vi "transfer function.vi"() -> ()   [LabVIEW 2016]
uses:
  <vilib>/DAQmx/write.llb/DAQmx Write (Analog Wfm 1Chan NSamp).vi
  <vilib>/DAQmx/read.llb/DAQmx Read (Analog Wfm 1Chan NSamp).vi
  <vilib>/DAQmx/create/channels.llb/DAQmx Create Channel (AO-Voltage-Basic).vi
  <vilib>/DAQmx/create/channels.llb/DAQmx Create Channel (AI-Voltage-Basic).vi
  <vilib>/DAQmx/configure/timing.llb/DAQmx Timing (Sample Clock).vi
  <vilib>/DAQmx/miscellaneous.llb/DAQmx Fill In Error Info.vi
  <vilib>/DAQmx/configure/trigger.llb/DAQmx Start Trigger (Digital Edge).vi
  <vilib>/Waveform/WDTFileIO.llb/Export Waveforms To Spreadsheet File (1D).vi
  <vilib>/measure/NI_MABase.lvlib
  <resource>/objmgr/daqmx.rc
panel:
  in  "File Name":string
  in  "Number of steps":i32
  in  "frequency stop":dbl=10.0 format="%0.2p"
  in  "file path (dialog if empty)":path
  out "Waveform Graph 2":waveform(dbl)(graph)
  in  "number of periods":dbl
  in  "amplitude":dbl=1.0 format="%0.2p"
  in  "frequency start":dbl=10.0 format="%0.2p"
  out "Waveform Graph":waveform(dbl)[](graph)
  out "number of samples written per channel":u32
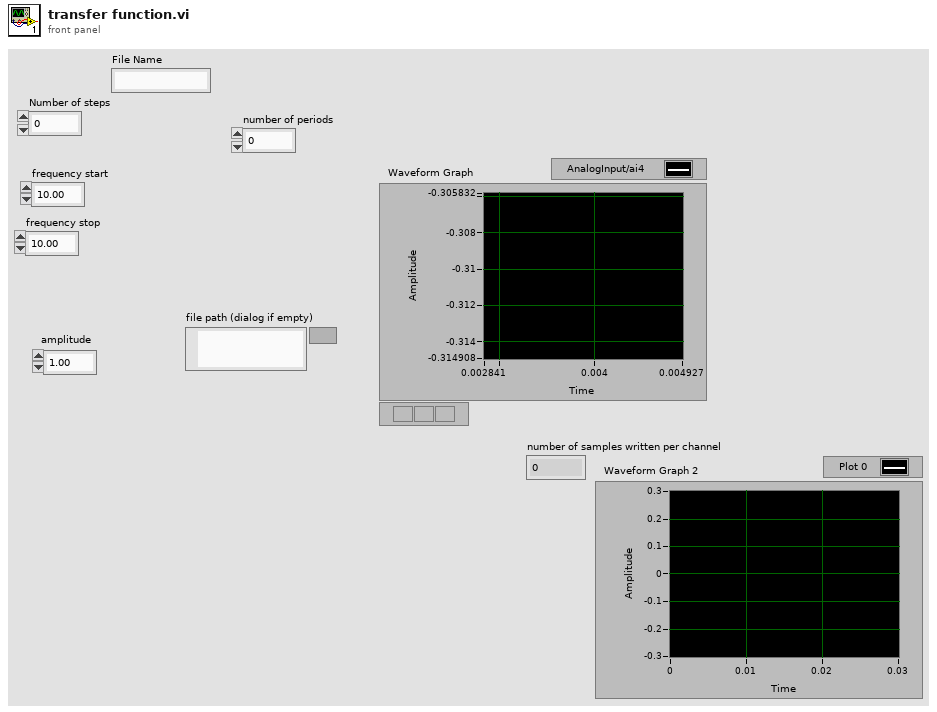
[diagram p1: front panel]
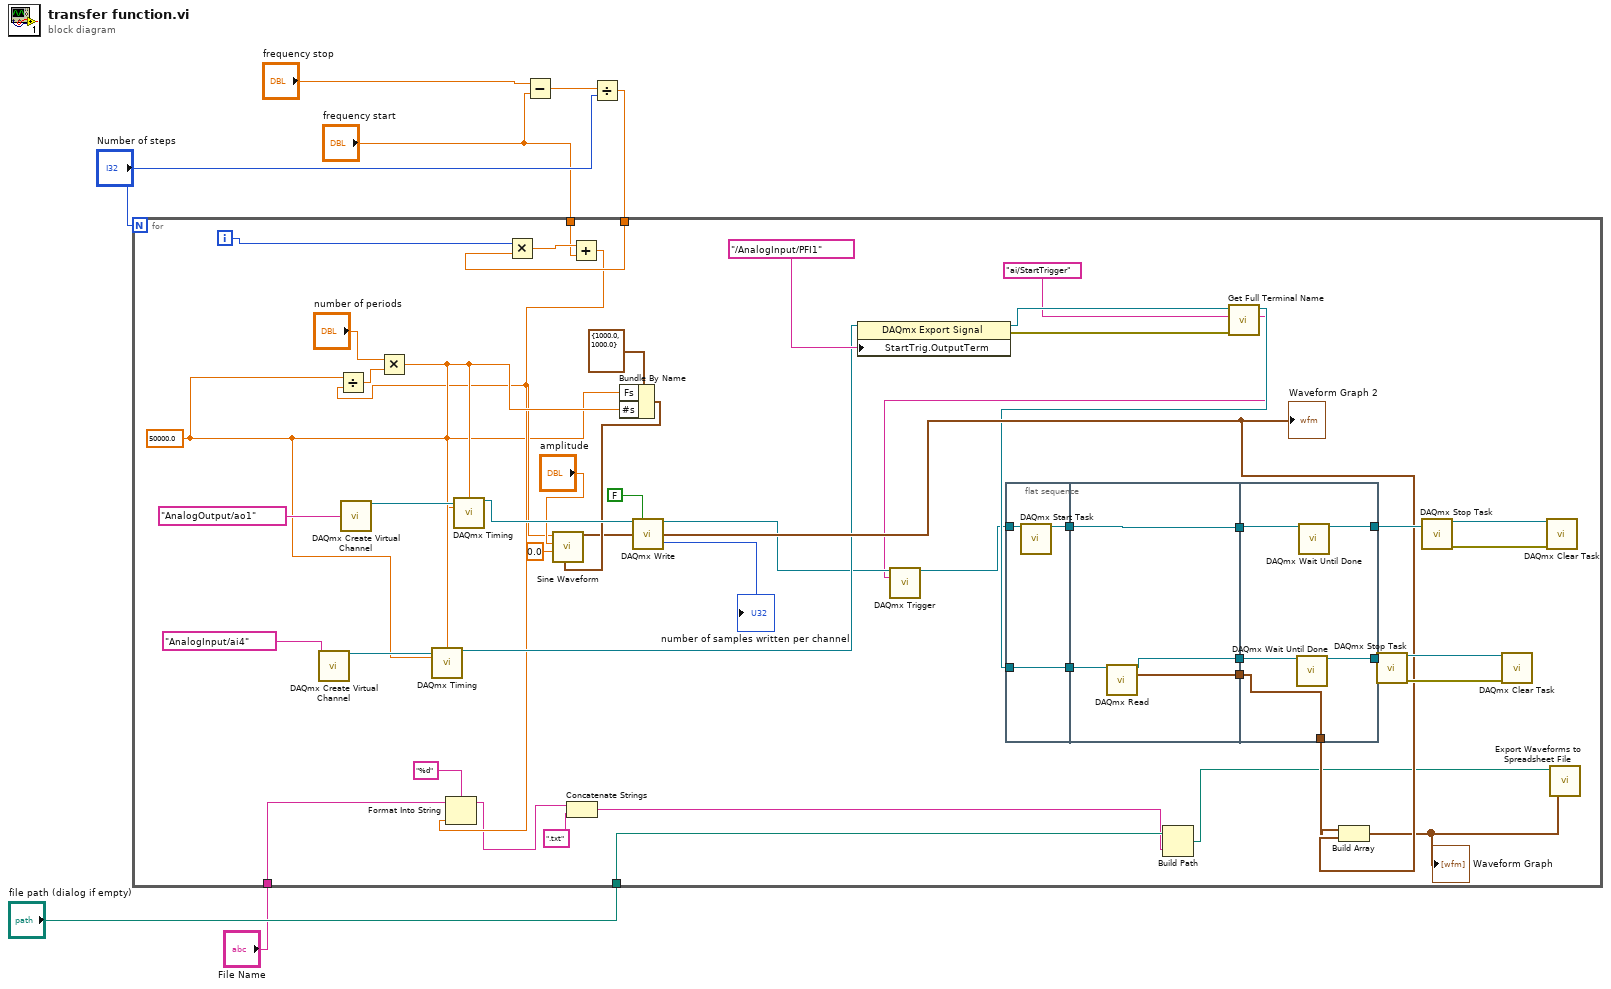
[diagram p0: block diagram]
diagram:
  n1 = Subtract(x="frequency stop", y="frequency start") -> (x-y=w7:dbl)
  n2 = Divide(x=w7, y="Number of steps") -> (x/y=w5:dbl)
  n3 = for {
    N: "Number of steps" -> [_]
    tunnel: w5 -> [w19]
    tunnel: "frequency start" -> [w17]
    tunnel: "file path (dialog if empty)" -> [w16]
    tunnel: "File Name" -> [w15]
    i -> [w20]
    w8 = 50000.0 ("rate")
    n4 = call-poly <vilib>:"DAQmx Create Virtual Channel.vi"("physical channels"=tag "AnalogInput/ai4") -> ("task out"=w45:refnum<k21>)  [unwired: 13 in, 1 out]
    n5 = call-poly <vilib>:"DAQmx Create Virtual Channel.vi"("physical channels"=tag "AnalogOutput/ao1") -> ("task out"=w50:refnum<k21>)  [unwired: 13 in, 1 out]
    n6 = Multiply(x=w20, y=w19) -> (x*y=w18:dbl)
    n7 = Add(x=w18, y=w17) -> (x+y=w14:dbl)
    n8 = Divide(x=w8, y=w14) -> (x/y=w37:dbl)
    n9 = Multiply(x="number of periods", y=w37) -> (x*y=w34:dbl)
    n10 = call-poly <vilib>:"DAQmx Timing.vi"("task/channels in"=w45, "samples per channel"=w34, "rate"=w8) -> ("task out"=w27:refnum<k21>)  [unwired: 11 in, 1 out]
    n11 = Format Into String(format string="%d", initial string=w15, w14) -> (resulting string=w11:string)  [unwired: 1 in, 1 out]
    n12 = call-poly <vilib>:"DAQmx Timing.vi"("task/channels in"=w50, "samples per channel"=w34, "rate"=w8) -> ("task out"=w49:refnum<k21>)  [unwired: 11 in, 1 out]
    n13 = Concatenate Strings(w11, ".txt" ("string")) -> (w10:string)
    n14 = Bundle By Name(cluster=cluster{"Fs":dbl, "#s":dbl} {"Fs"=1000.0, "#s"=1000.0} ("sampling info"), "Fs"=w8, "#s"=w34) -> (w35:cluster{"Fs":dbl, "#s":dbl})
    n15 = call <vilib>:"Sine Waveform.vi"("sampling info"=w35, "phase"=0.0, "amplitude"="amplitude", "frequency"=w14) -> ("signal out"=w32:waveform(dbl))  [unwired: 6 in, 1 out]
    "Waveform Graph 2" <- w32
    n16 = call-poly <vilib>:"DAQmx Write.vi"("task/channels in"=w49, "auto start"=FALSE, "data"=w32) -> ("task out"=w25:refnum<k21>, "number of samples written per channel"=→"number of samples written per channel":u32)  [unwired: 10 in, 1 out]
    n17 = property class="DAQmx Export Signal"(reference=w27, "StartTrig.OutputTerm"=tag "/AnalogInput/PFI1") -> (reference out=w29:refnum<k21>, error out=w30:errorcluster)  [unwired: 1 in]
    n18 = flat-sequence {
      tunnel: w24 -> [w60]
      tunnel: [w59] -> w57
      tunnel: w26 -> [w58]
      tunnel: [w58] -> w56
      tunnel: w57 -> [w64]
      tunnel: w56 -> [w63]
      tunnel: [w64] -> w55
      tunnel: [w62] -> w54
      tunnel: [w61] -> w53
      tunnel: w55 -> [w69]
      tunnel: [w68] -> w43
      tunnel: [w67] -> w40
      tunnel: w54 -> [w66]
      tunnel: [w65] -> w33
      tunnel: w53 -> [w65]
      frame #0 {
        n19 = call <vilib>:"DAQmx Start Task.vi"("task/channels in"=w60) -> ("task out"=w59:refnum<k21>)  [unwired: 13 in, 1 out]
      }
      frame #1 {
        n20 = call-poly <vilib>:"DAQmx Read.vi"("task/channels in"=w63) -> ("task out"=w62:refnum<k21>, "data"=w61:waveform(dbl))  [unwired: 12 in, 1 out]
      }
      frame #2 {
        n21 = call <vilib>:"DAQmx Wait Until Done.vi"("task/channels in"=w66) -> ("task out"=w67:refnum<k21>)  [unwired: 13 in, 1 out]
        n22 = call <vilib>:"DAQmx Wait Until Done.vi"("task/channels in"=w69) -> ("task out"=w68:refnum<k21>)  [unwired: 13 in, 1 out]
      }
    }
    n23 = Build Path(base path=w16, name or relative path=w10) -> (appended path=w13:path)
    n24 = call "Get Full Terminal Name.vi"("error in (no error)"=w30, "Local Terminal Name"="ai/StartTrigger", "task/channels in"=w29) -> ("Terminal Name with Device Prefix"=w23:tag, "task out"=w26:refnum<k21>)  [unwired: 6 in, 1 out]
    n25 = call-poly <vilib>:"DAQmx Trigger.vi"("task/channels in"=w25, "source"=w23) -> ("task out"=w24:refnum<k21>)  [unwired: 12 in, 1 out]
    n26 = Build Array(w33, w32) -> (w22:waveform(dbl)[])
    "Waveform Graph" <- w22
    n27 = call <vilib>:"DAQmx Stop Task.vi"("task/channels in"=w40) -> ("task out"=w42:refnum<k21>, "error out"=w41:errorcluster)  [unwired: 13 in]
    n28 = call <vilib>:"DAQmx Stop Task.vi"("task/channels in"=w43) -> ("task out"=w47:refnum<k21>, "error out"=w46:errorcluster)  [unwired: 13 in]
    n29 = call <vilib>:"DAQmx Clear Task.vi"("task in"=w42, "error in"=w41) -> ()  [unwired: 13 in, 1 out]
    n30 = call <vilib>:"DAQmx Clear Task.vi"("task in"=w47, "error in"=w46) -> ()  [unwired: 13 in, 1 out]
    n31 = call-poly <vilib>:"Export Waveforms to Spreadsheet File.vi"("waveforms"=w22, "file path (dialog if empty)"=w13) -> ()  [unwired: 8 in, 2 out]
  }
